vi "FTW-Endpoint-Connect.vi"(0 "FTW ØMQ Endpoint":refnum<class "FTW-Endpoint-ZMQ.lvclass">, 5 "Endpoint Address":T1, 11 "error in":errorcluster) -> (4 "FTW ØMQ Endpoint out":refnum<class "FTW-Endpoint-ZMQ.lvclass">, 15 "error out":errorcluster)   [LabVIEW 2012, in "FTW-Endpoint-ZMQ.lvclass"]
uses:
  FTW-Endpoint-ZMQ.lvclass
  Utility/FTW-Actor-Address.ctl
  FTW-Endpoint-ZMQ.lvclass/FTW-Endpoint-ZMQ.ctl
  FTW-Actor.lvlib
panel:
  # "Inputs"
  # "Outputs"
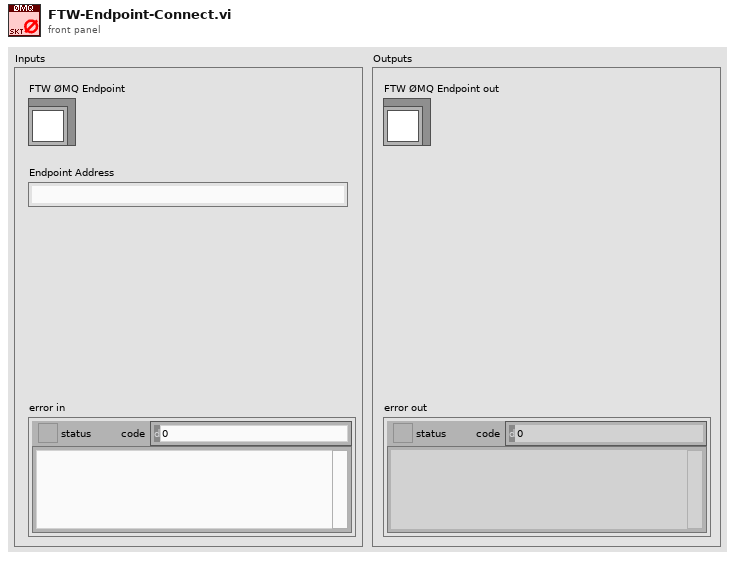
[diagram p1: front panel]
types:
  T1 = typedef "FTW-Actor.lvlib/FTW-Actor-Address.ctl" = string
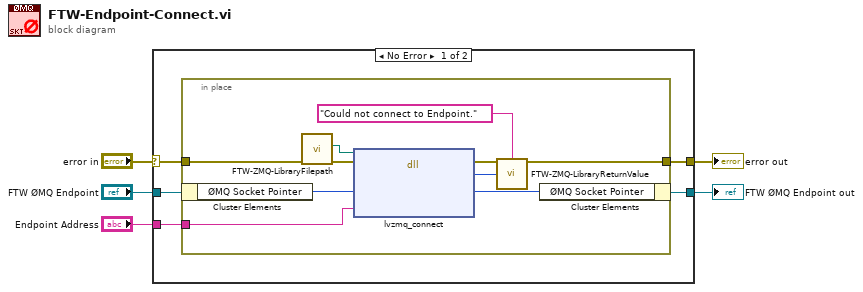
[diagram p0: block diagram]
diagram:
  n1 = case shown="No Error" "error in" {
    selector: "error in" -> [w8 w21]
    tunnel: "FTW ØMQ Endpoint" -> [w10 w22]
    tunnel: [w7 w21] -> w4
    tunnel: [w9 w22] -> w3
    tunnel: "Endpoint Address" -> [w6 _]
    frame No Error {
      n2 = in-place {
        in-place-border: w8 -> [w19]
        in-place-border: [w18] -> w7
        in-place-border: w6 -> [w17]
        n3 = in-place-cluster #1(w10) -> ("ØMQ Socket Pointer"=w20:u64)
        n4 = call "FTW-ZMQ-LibraryFilepath.vi"("error in"=w19) -> ("error out"=w12:errorcluster, "FTW-ZMQ Library Filepath"=w11:path)  [unwired: 8 in, 1 out]
        n5 = dll-call lib="?" fn="lvzmq_connect" ("zmq_labview.dll:lvzmq_bind")(path in=w11, error in=w12, "Socket Pointer"=w20, "Endpoint"=w17) -> (error out=w15:errorcluster, "Return Value"=w14:i32, "Socket Pointer"=w16:u64)  [unwired: 2 in, 1 out]
        n6 = call "FTW-ZMQ-LibraryReturnValue.vi"("error in"=w15, "Error Message"="Could not connect to Endpoint.", "Return Value"=w14) -> ("error out"=w18:errorcluster)  [unwired: 12 in]
        n7 = in-place-cluster #1("ØMQ Socket Pointer"=w16) -> (w9:refnum<class "FTW-Endpoint-ZMQ.lvclass">)
      }
    }
    frame Error {
    }
  }
  "error out" <- w4
  "FTW ØMQ Endpoint out" <- w3
